vi "delay one channel.vi"(9 "Delay":u8 max=5 step=1, 10 "Wet/Dry":dbl, 11 "Audio In":i16[](array[numeric])) -> (3 "Audio Out":i16[](array[numeric]))   [LabVIEW 2014]
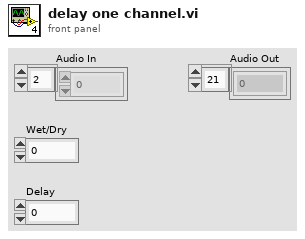
[diagram p1: front panel]
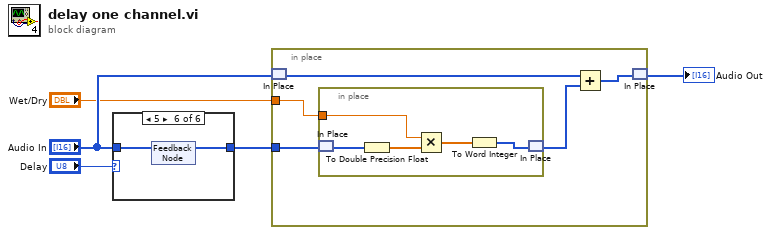
[diagram p0: block diagram]
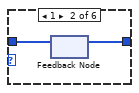
[diagram p3: hidden frame]
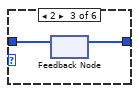
[diagram p4: hidden frame]
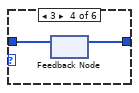
[diagram p5: hidden frame]
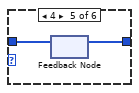
[diagram p6: hidden frame]
diagram:
  n1 = case shown="5" "Delay" {
    tunnel: "Audio In" -> [w6 w8 w10 w12 w14 w16]
    tunnel: [w6 w7 w9 w11 w13 w15] -> w3
    frame 0, Default {
    }
    frame 1 {
      n2 = feedback-in #1(w8) -> ()
      n3 = feedback #1() -> (w7:i16[])  [unwired: 1 in]
    }
    frame 2 {
      n4 = feedback-in #2(w10) -> ()
      n5 = feedback #2() -> (w9:i16[])  [unwired: 1 in]
    }
    frame 3 {
      n6 = feedback-in #3(w12) -> ()
      n7 = feedback #3() -> (w11:i16[])  [unwired: 1 in]
    }
    frame 4 {
      n8 = feedback-in #4(w14) -> ()
      n9 = feedback #4() -> (w13:i16[])  [unwired: 1 in]
    }
    frame 5 {
      n10 = feedback-in #5(w16) -> ()
      n11 = feedback #5() -> (w15:i16[])  [unwired: 1 in]
    }
  }
  n12 = in-place {
    in-place-border: w3 -> [w18]
    in-place-border: "Wet/Dry" -> [w19]
    n13 = in-place-match #6("Audio In") -> (w21:i16[])
    n14 = in-place {
      in-place-border: w19 -> [w24]
      n15 = in-place-match #7(w18) -> (w23:i16[])
      n16 = To Double Precision Float(number=w23) -> (double precision float=w26:dbl[])
      n17 = Multiply(x=w24, y=w26) -> (x*y=w25:dbl[])
      n18 = To Word Integer(number=w25) -> (16bit integer=w22:i16[])
      n19 = in-place-match #7(w22) -> (w17:i16[])
    }
    n20 = Add(x=w21, y=w17) -> (x+y=w20:i16[])
    n21 = in-place-match #6(w20) -> (→"Audio Out":i16[])
  }
